vi "Stop Core.vi"(10 "final error code":i32, 11 "TcpServer in":refnum<class "TcpServer.lvclass">) -> (3 "TcpServer out":refnum<class "TcpServer.lvclass">)   [LabVIEW 2022 SP3, in "TcpServer.lvlib" / "TcpServer.lvclass"]
doc: "(<B>Filename</B>: Actor Framework.lvlib:Actor.lvclass:Stop Core.vi)\n\nDefines what the actor does before it stops. Use the <B>final error code</B> input to determine whether the actor shut down in response to an error.\n\nBy default, this method does nothing. A descendant class may override it to define behavior, such as shutting down any processes the actor initiated in its override of the Actor Core method."
uses:
  TcpServer.lvclass
  TcpServer.lvclass/TcpServer.ctl
  TcpSocket/Source/TcpSocket/TcpServer/TcpServer.lvclass
  LoggingActor/Source/LoggingActor/LoggingActor/LoggingActor.lvclass
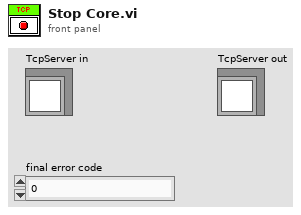
[diagram p1: front panel]
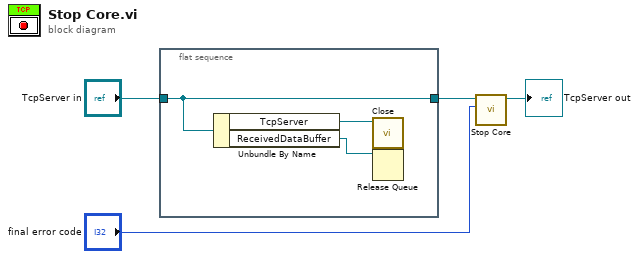
[diagram p0: block diagram]
diagram:
  n1 = flat-sequence {
    tunnel: "TcpServer in" -> [w6]
    tunnel: [w6] -> w1
    frame #0 {
      n2 = Unbundle By Name(w6) -> ("TcpServer"=w7:refnum<class "TcpServer.lvclass">, "ReceivedDataBuffer"=w5:refnum<queue>)
      n3 = call-dynamic "Close.vi"("TcpSocket in"=w7) -> ()  [unwired: 10 in, 1 out]
      n4 = Release Queue(queue=w5) -> ()  [unwired: 2 in, 3 out]
    }
  }
  n5 = call-parent "Stop Core.vi"("final error code"="final error code", "LoggingActor in"=w1) -> ("LoggingActor out"=→"TcpServer out":refnum<class "TcpServer.lvclass">)  [unwired: 9 in]
